vi "RNN.vi"(3 "Input 2":u16, 4 "Input 1":u16, 5 "Weights":sgl[](array[numeric])) -> (0 "Downwards":u16, 1 "Still":u16, 2 "Upwards":u16)   [LabVIEW 2020]
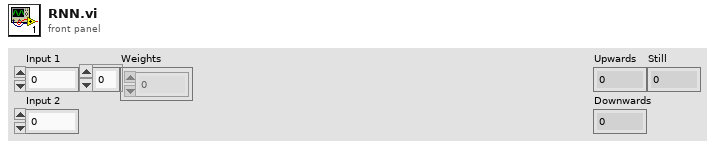
[diagram p1: front panel]
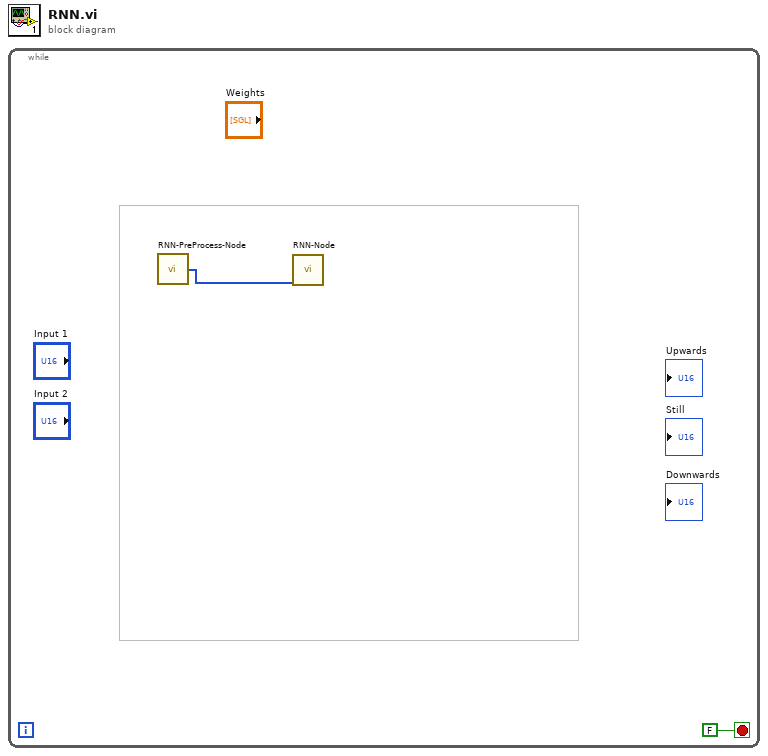
[diagram p0: block diagram]
diagram:
  n1 = while {
    stop <- FALSE stop-if-true
    n2 = call "RNN-PreProcess-Node.vi"() -> ("Output"=w1:i16[])  [unwired: 6 in]
    n3 = call "RNN-Node.vi"("Input_Array"=w1) -> ()  [unwired: 4 in, 1 out]
  }
